vi "Write Motors.vi"(8 "error in (no error)":errorcluster, 10 "Actor Framework:Message Enqueuer":refnum<class "Message Enqueuer.lvclass">, 11 "Receive Updates from Motors with Encoders in":refnum<class "Receive Updates from Motors with Encoders.lvclass">) -> (0 "error out":errorcluster, 3 "Receive Updates from Motors with Encoders out":refnum<class "Receive Updates from Motors with Encoders.lvclass">)   [LabVIEW 2014, in "Comp Motors with Encoders.lvlib" / "Receive Updates from Motors with Encoders.lvclass"]
uses:
  Receive Updates from Motors with Encoders.lvclass
  <vilib>/ActorFramework/Message Enqueuer/Message Enqueuer.lvclass
  Receive Updates from Motors with Encoders.lvclass/Receive Updates from Motors with Encoders.ctl
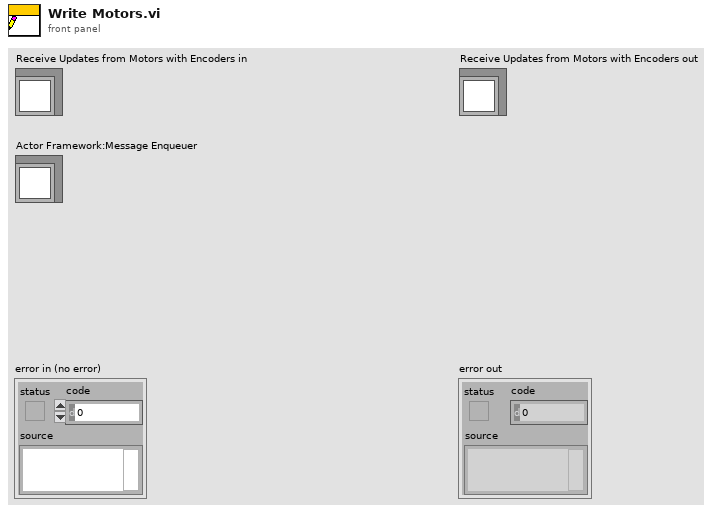
[diagram p1: front panel]
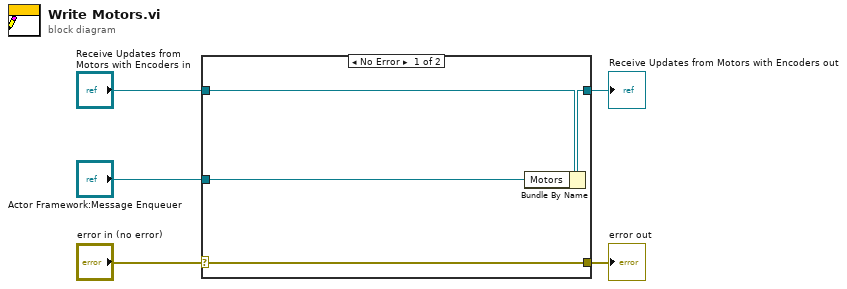
[diagram p0: block diagram]
diagram:
  n1 = case shown="No Error" "error in (no error)" {
    selector: "error in (no error)" -> [w9 w10]
    tunnel: [w9 w10] -> w4
    tunnel: [w7 w11] -> w2
    tunnel: "Receive Updates from Motors with Encoders in" -> [w8 w11]
    tunnel: "Actor Framework:Message Enqueuer" -> [w6 _]
    frame No Error {
      n2 = Bundle By Name(cluster=w8, "Motors"=w6) -> (w7:refnum<class "Receive Updates from Motors with Encoders.lvclass">)
    }
    frame Error {
    }
  }
  "error out" <- w4
  "Receive Updates from Motors with Encoders out" <- w2
